vi "week03_Ex3.vi"() -> ()   [LabVIEW 2017]
panel:
  out "x != y?":bool
  out "all lower case string":string
  out "substring":string
  out "length 2":i32
  out "trimmed string":string
  out "length":i32
  in  "String 1":string
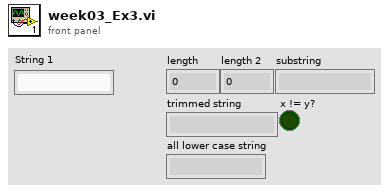
[diagram p1: front panel]
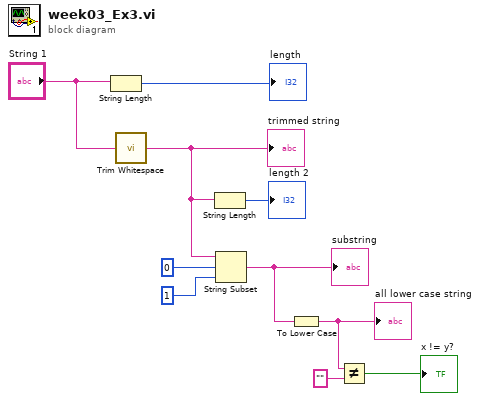
[diagram p0: block diagram]
diagram:
  n1 = String Length(string="String 1") -> (length=→"length":i32)
  n2 = call <vilib>:"Trim Whitespace.vi"("string"="String 1") -> ("trimmed string"=w7:string)  [unwired: 1 in]
  "trimmed string" <- w7
  n3 = String Length(string=w7) -> (length=→"length 2":i32)
  n4 = String Subset(string=w7, offset (0)=0, length (rest)=1 ("length (rest)")) -> (substring=w4:string)
  "substring" <- w4
  n5 = To Lower Case(string=w4) -> (all lower case string=w3:string)
  "all lower case string" <- w3
  n6 = Not Equal?(x=w3, y="") -> (x != y?=→"x != y?":bool)
